vi "Add Entity to Container.vi"(7 "Project":string, 8 "error in (no error)":errorcluster, 9 "Library":bool, 10 "Container":string, 11 "Entity Path":path) -> (0 "error out":errorcluster, 3 "Entity Class":refnum<vi>)   [LabVIEW 2020, in "Conditum-Tools.lvlib" / "Entity Editor.lvclass"]
uses:
  Entity Editor.lvclass
  Entity Editor.lvclass/Entity Editor.ctl
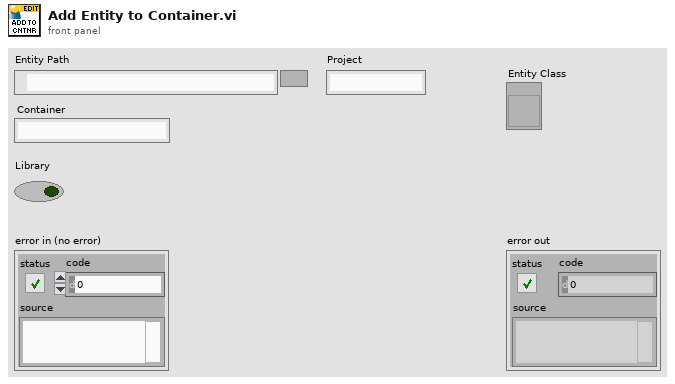
[diagram p1: front panel]
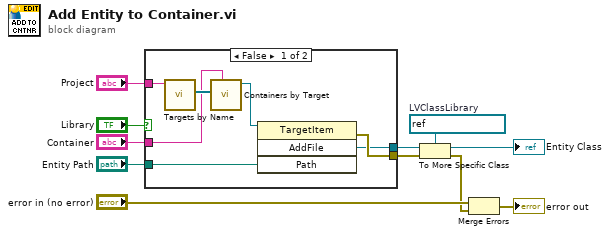
[diagram p0: block diagram]
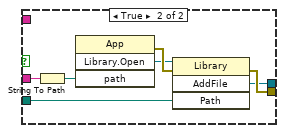
[diagram p2: hidden frame]
diagram:
  w1 = refnum<vi> refnum  # LVClassLibrary
  n1 = case shown="False" "Library" {
    tunnel: "Entity Path" -> [w12 w23]
    tunnel: "Container" -> [w15 w22]
    tunnel: "Project" -> [w16 _]
    tunnel: [w13 w19] -> w5
    tunnel: [w18 w24] -> w4
    frame False {
      n2 = call "Targets by Name.vi"("Project Name"=w16) -> ("Targets"=w17:refnum<vi>[])  [unwired: 9 in, 1 out]
      n3 = call "Containers by Target.vi"("Target Name"=w15, "Targets"=w17) -> ("Target"=w14:refnum<vi>)  [unwired: 7 in, 2 out]
      n4 = invoke class="TargetItem" method="AddFile"(reference=w14, "Path"=w12) -> (error out=w18:errorcluster, "AddFile"=w13:refnum<vi>)  [unwired: 2 in, 2 out]
    }
    frame True {
      n5 = String To Path(string=w22) -> (path=w21:path)
      n6 = invoke class="App" method="Library.Open"("path"=w21) -> (error out=w25:errorcluster, "Open Library"=w20:refnum<vi>)  [unwired: 3 in, 2 out]
      n7 = invoke class="Library" method="AddFile"(reference=w20, error in=w25, "Path"=w23) -> (error out=w24:errorcluster, "AddFile"=w19:refnum<vi>)  [unwired: 1 in, 2 out]
    }
  }
  n8 = To More Specific Class(target class=w1, reference=w5, error in=w4) -> (specific class reference=→"Entity Class":refnum<vi>, error out=w2:errorcluster)
  n9 = Merge Errors("error in (no error)", w2) -> (→"error out":errorcluster)
